vi "Process.vi"(8 "error in":errorcluster, 11 "Plugin in":refnum<class "Output Sequencer.lvclass">) -> (0 "error out":errorcluster, 3 "Plugin out":refnum<class "Output Sequencer.lvclass">)   [LabVIEW 2024, in "Output Sequencer.lvlib" / "Output Sequencer.lvclass"]
uses:
  Output Sequencer.lvclass
  Output Sequencer.lvclass/Output Sequencer.ctl
  Types/Sequencer State.ctl
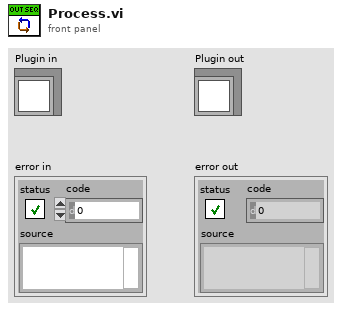
[diagram p1: front panel]
types:
  T1 = typedef "Output Sequencer.lvlib/Output Sequencer.lvclass/Sequencer State.ctl" = enum16{"Error", "Initialize", "Prepare channels", "Wait for test", "Wait for %.1f sec", "Wait for trigger", "Stop condition", "Wait for resume", "Running", "Paused", "No valid step", "Stopped"}
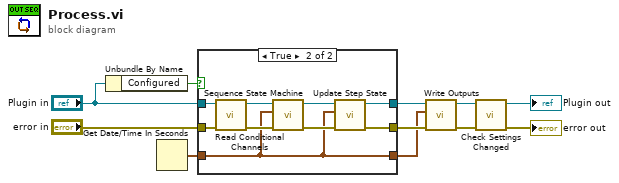
[diagram p0: block diagram]
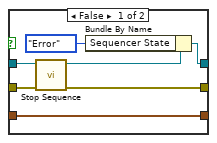
[diagram p2: hidden frame]
diagram:
  n1 = Unbundle By Name("Plugin in") -> ("Configured"=w1:bool)
  n2 = Get Date/Time In Seconds() -> (seconds since 1Jan1904=w8:timestamp)
  n3 = case shown="True" w1 {
    tunnel: "Plugin in" -> [w16 w27]
    tunnel: "error in" -> [w17 w26]
    tunnel: w8 -> [w18 w19]
    tunnel: [w13 w21] -> w7
    tunnel: [w14 w20] -> w6
    tunnel: [w18 w19] -> w3
    frame False {
      n4 = call "Stop Sequence.vi"("error in (no error)"=w17, "Output Sequencer in"=w16) -> ("error out"=w14:errorcluster, "Output Sequencer out"=w15:refnum<class "Output Sequencer.lvclass">)  [unwired: 7 in, 1 out]
      n5 = Bundle By Name(cluster=w15, "Sequencer State"=Sequencer_State."Error" ("State.Sequencer State")) -> (w13:refnum<class "Output Sequencer.lvclass">)
    }
    frame True {
      n6 = call "Read Conditional Channels.vi"("error in (no error)"=w26, "Output Sequencer in"=w27) -> ("error out"=w24:errorcluster, "Output Sequencer out"=w25:refnum<class "Output Sequencer.lvclass">)  [unwired: 8 in]
      n7 = call "Sequence State Machine.vi"("error in (no error)"=w24, "Current time"=w19, "Output Sequencer in"=w25) -> ("error out"=w22:errorcluster, "Output Sequencer out"=w23:refnum<class "Output Sequencer.lvclass">)  [unwired: 7 in]
      n8 = call "Update Step State.vi"("error in (no error)"=w22, "Current Time"=w19, "Output Sequencer in"=w23) -> ("error out"=w20:errorcluster, "Output Sequencer out"=w21:refnum<class "Output Sequencer.lvclass">)  [unwired: 7 in]
    }
  }
  n9 = call "Write Outputs.vi"("error in (no error)"=w6, "Current time"=w3, "Output Sequencer in"=w7) -> ("error out"=w4:errorcluster, "Output Sequencer out"=w5:refnum<class "Output Sequencer.lvclass">)  [unwired: 7 in]
  n10 = call "Check Settings Changed.vi"("error in (no error)"=w4, "Output Sequencer in"=w5) -> ("error out"=→"error out":errorcluster, "Output Sequencer out"=→"Plugin out":refnum<class "Output Sequencer.lvclass">)  [unwired: 8 in]
